vi "BufferedRunQueue.vi"() -> ()   [LabVIEW 2010]
panel:
  in  "task":i32=1
  out "error out":errorcluster
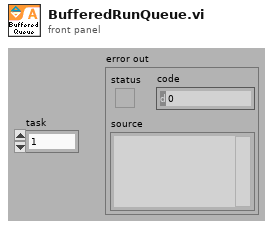
[diagram p1: front panel]
types:
  T1 = enum16{"open", "replace", "create", "open or create", "replace or create", "replace or create with confirmation"}
  T2 = typedef "TaskStatus.ctl" = cluster{"Task Status0 (num)":i32, "Task Status0 (bits)":cluster{"CallbackHoldActive":bool, "CallbackResponding":bool, "CannedFunctionExecuting":bool, "CornerRounding":bool, "FeedHoldActive":bool, "ImmediateConcurrent":bool, "ImmediateExecuting":bool, "InterruptMotionActive":bool, "JoystickActive":bool, "JoystickLowSpeedActive":bool, "None":bool, "PendingAxesStop":bool, "ProbeCycle":bool, "ProgramAssociated":bool, "ProgramControlRestricted":bool, "ProgramReset":bool, "Retrace":bool, "ReturnMotionExecuting":bool, "SingleStepInto":bool, "SingleStepOver":bool, "SoftHomeActive":bool, "SoftwareESTOPActive":bool, "SpindleActive0":bool, "SpindleActive1":bool, "SpindleActive2":bool, "SpindleActive3":bool}, "Task Status0 (str)":string, "Task Status1 (num)":i32, "Task Status1 (bits)":cluster{"AsyncSMCMotionAbortPending":bool, "CannedFunctionPending":bool, "CutterOffsetsDisabling":bool, "CutterOffsetsEnablingNegative":bool, "CutterOffsetsEnablingPositive":bool, "CutterRadiusDisabling":bool, "CutterRadiusEnabling":bool, "FeedHeldAxesStopped":bool, "GalvoIFVDeactivationPending":bool, "IFOVBufferHold":bool, "Interrupted":bool, "MotionModeAbsOffsets":bool, "MSOChange":bool, "NoMFOFloor":bool, "None":bool, "OnGosubPending":bool, "ProgramStopPending":bool, "RetraceRequested":bool, "SpindleFeedHeld":bool}, "Task Status1 (str)":string, "Task Status2 (num)":i32, "Task Status2 (bits)":cluster{"Coord1Plane1":bool, "Coord1Plane2":bool, "Coord1Plane3":bool, "Coord2Plane1":bool, "Coord2Plane2":bool, "Coord2Plane3":bool, "CutterOffsetsActiveNeg":bool, "CutterOffsetsActivePos":bool, "CutterRadiusActiveLeft":bool, "CutterRadiusActiveRight":bool, "LimitFeedRateActive":bool, "LimitMFOActive":bool, "MirrorActive":bool, "MotionContinuousActive":bool, "MotionFiber":bool, "MotionModeCCW":bool, "MotionModeCoordinated":bool, "MotionModeCW":bool, "MotionModeRapid":bool, "MotionPVT":bool, "None":bool, "NormalcyActiveLeft":bool, "NormalcyActiveRight":bool, "NormalcyAlignment":bool, "OffsetFixtureActive":bool, "ProfileActive":bool, "RotationActive":bool, "RThetaCylindricalActive":bool, "RThetaPolarActive":bool, "ScalingActive":bool}, "Task Status2 (str)":string, "Task Mode (num)":i32, "Task Mode (bits)":cluster{"Absolute":bool, "AccelModeRate":bool, "AccelTypeLinear":bool, "AccelTypeScurve":bool, "AutoMode":bool, "BlockDelete":bool, "BlockDelete2":bool, "DecelModeRate":bool, "DecelTypeLinear":bool, "DecelTypeScurve":bool, "InverseCircular":bool, "InverseDominance":bool, "MFOActiveOnJog":bool, "MFOLock":bool, "Minutes":bool, "MotionContinuous":bool, "MSOLock":bool, "None":bool, "OptionalPause":bool, "OverMode":bool, "ProgramFeedRateMPU":bool, "ProgramFeedRateUPR":bool, "Secondary":bool, "SpindleStopOnProgramHalt":bool, "WaitAuto":bool, "WaitForInPos":bool}, "Task Mode (str)":string, "Queue Status (num)":i32, "Queue Status (bits)":cluster{"None":bool, "QueueBufferEmpty":bool, "QueueBufferFull":bool, "QueueBufferPaused":bool, "QueueBufferStarted":bool, "QueueLargeProgramExecuting":bool, "QueueModeActive":bool}, "Queue Status (str)":string, "Task State":i32}
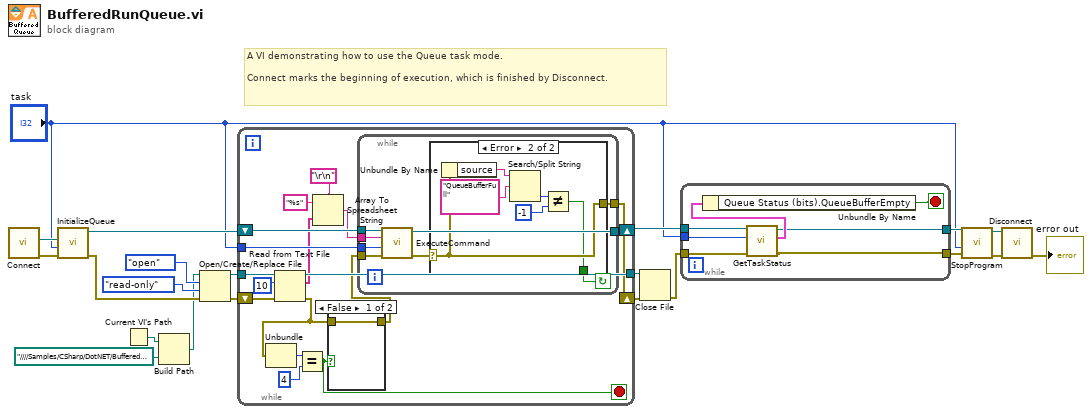
[diagram p0: block diagram]
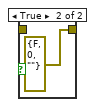
[diagram p2: hidden frame]
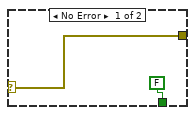
[diagram p3: hidden frame]
diagram:
  # "A VI demonstrating how to use the Queue task mode.\n\nConnect marks the beginning of execution, which is finished by Disconnect."
  n1 = call "Connect.vi"() -> ("error out"=w21:errorcluster, "controller"=w20:refnum<k24>)  [unwired: 10 in]
  n2 = call "InitializeQueue.vi"("error in (no error)"=w21, "taskId"="task", "controller in"=w20) -> ("error out"=w4:errorcluster, "controller out"=w15:refnum<k24>)  [unwired: 7 in]
  n3 = Current VI's Path() -> (path=w3:path)
  n4 = Build Path(base path=w3, name or relative path=path "../../../../Samples/CSharp/DotNET/Buffered Run Queue/file.txt") -> (appended path=w1:path)
  n5 = Open/Create/Replace File(file path (use dialog)=w1, error in=w4, operation (0:open)=T1."open", access (0:read/write)=enum16{"read/write", "read-only", "write-only"}."read-only") -> (refnum out=w5:refnum<file>, error out=w6:errorcluster)  [unwired: 2 in, 1 out]
  n6 = while {
    tunnel: "task" -> [w38]
    shift-right: [w32] -> w9
    shift-left: w6 -> [w35]
    shift-right: [w36] -> w19
    shift-left: w15 -> [w37]
    tunnel: w5 -> [w34]
    tunnel: [w33] -> w8
    stop <- w26 stop-if-true
    n7 = Read from Text File(file (use dialog)=w34, count=10, error in=w35) -> (refnum out=w33:refnum<file>, text=w25:string[], error out=w29:errorcluster)  [unwired: 1 in, 1 out]
    n8 = Unbundle(w29) -> ("code"=w30:i32)  [unwired: 2 out]
    n9 = Equal?(x=w30, y=4 ("x")) -> (x = y?=w26:bool)
    n10 = Array To Spreadsheet String(delimiter (Tab)="\r\n", array=w25, 3:"%s" ("format string")) -> (spreadsheet string=w22:string)
    n11 = case shown="False" w26 {
      tunnel: w29 -> [w39 _]
      tunnel: [w39 errorcluster {"status"=FALSE, "code"=0, "source"=""} ("error out")] -> w28
      frame False {
      }
      frame True {
      }
    }
    n12 = while {
      tunnel: w28 -> [w46]
      tunnel: w38 -> [w44]
      tunnel: [w47] -> w32
      tunnel: w37 -> [w43]
      tunnel: w22 -> [w42]
      tunnel: [w41] -> w36
      stop <- w48 continue-if-true
      n13 = call "ExecuteCommand.vi"("error in (no error)"=w46, "taskId"=w44, "Command Code"=w42, "controller in"=w43) -> ("error out"=w45:errorcluster, "controller out"=w41:refnum<k24>)  [unwired: 5 in, 1 out]
      n14 = case shown="Error" w45 {
        selector: w45 -> [w49 w56]
        tunnel: [FALSE w51] -> w48
        tunnel: [w49 w56] -> w47
        frame No Error {
        }
        frame Error {
          n15 = Unbundle By Name(w56) -> ("source"=w55:string)
          n16 = Search/Split String(string=w55, search string/char (-)="QueueBufferFull" ("true string")) -> (offset of match=w53:i32)  [unwired: 1 in, 2 out]
          n17 = Not Equal?(x=w53, y=-1) -> (x != y?=w51:bool)
        }
      }
    }
  }
  n18 = Close File(refnum=w8, error in=w9) -> (error out=w7:errorcluster)  [unwired: 1 out]
  n19 = while {
    tunnel: w19 -> [w62]
    tunnel: "task" -> [w63]
    tunnel: w7 -> [w61]
    tunnel: [w58] -> w17
    tunnel: [w57] -> w16
    stop <- w59 stop-if-true
    n20 = call "GetTaskStatus.vi"("error in (no error)"=w61, "task"=w63, "controller in"=w62) -> ("error out"=w58:errorcluster, "task status"=w60:T2, "controller out"=w57:refnum<k24>)  [unwired: 6 in]
    n21 = Unbundle By Name(w60) -> ("Queue Status (bits).QueueBufferEmpty"=w59:bool)
  }
  n22 = call "StopProgram.vi"("error in (no error)"=w17, "taskId"="task", "controller in"=w16) -> ("error out"=w14:errorcluster, "controller out"=w13:refnum<k24>)  [unwired: 7 in]
  n23 = call "Disconnect.vi"("error in (no error)"=w14, "controller"=w13) -> ("error out"=→"error out":errorcluster)  [unwired: 9 in]
